vi "SaveReport(SubVI).vi"(8 "Error In":errorcluster, 9 "1D data":string[](array[string]), 10 "2D Data":string[][](array[string])=[[" ", " "]], 11 "FileName":string) -> (0 "Error Out":errorcluster)   [LabVIEW 2018, in "DS_Lib.lvlib" / "SRReportParser.lvlib"]
uses:
  SRReportParser.lvlib
  <vilib>/Utility/file.llb/Write Delimited Spreadsheet (string).vi
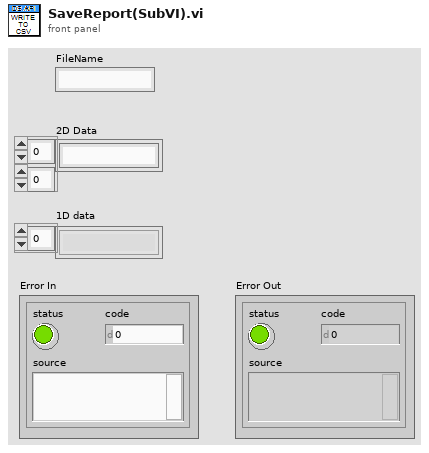
[diagram p1: front panel]
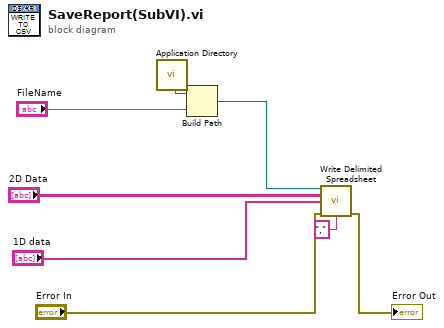
[diagram p0: block diagram]
diagram:
  n1 = call <vilib>:"Application Directory.vi"() -> ("Application Directory"=w8:path)
  n2 = Build Path(base path=w8, name or relative path="FileName") -> (appended path=w6:path)
  n3 = call-poly <vilib>:"Write Delimited Spreadsheet.vi"("file path (dialog if empty)"=w6, "2D data"="2D Data", "1D data"="1D data", "error in (no error)"="Error In", "delimiter (\\t)"="," ("delimiter (\\t)")) -> ("error out"=→"Error Out":errorcluster)  [unwired: 9 in, 1 out]
